vi "Get SLSC Modules By GUID.vi"(8 "error in (no error)":errorcluster, 10 "GUID":string, 11 "SLSC Chassis":u64) -> (0 "error out":errorcluster, 1 "Found":bool, 2 "SLSC Modules":u64[](array[numeric]), 3 "SLSC Chassis out":u64)   [LabVIEW 2017, in "VeriStand SLSC Scripting.lvlib"]
uses:
  VeriStand SLSC Scripting.lvlib
  NationalInstruments.VeriStand.SystemDefinitionAPI
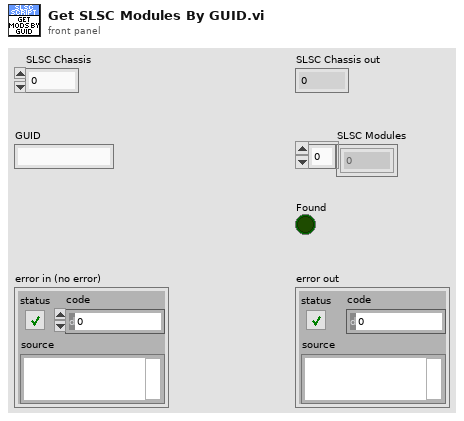
[diagram p1: front panel]
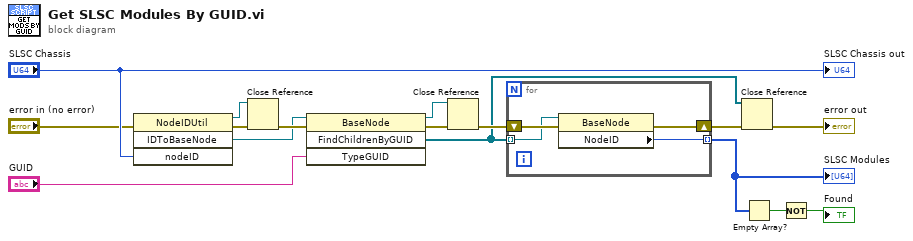
[diagram p0: block diagram]
diagram:
  n1 = invoke class="NodeIDUtil" method="IDToBaseNode"(error in="error in (no error)", "nodeID"="SLSC Chassis") -> (reference out=w15:refnum<k24>, error out=w16:errorcluster, "IDToBaseNode"=w8:refnum<k24>)  [unwired: 2 in, 1 out]
  n2 = Close Reference(reference=w15, error in (no error)=w16) -> (error out=w9:errorcluster)
  n3 = invoke class="BaseNode" method="FindChildrenByGUID"(reference=w8, error in=w9, "TypeGUID"="GUID") -> (reference out=w5:refnum<k24>, error out=w6:errorcluster, "FindChildrenByGUID"=w4:refnum<k24>[])  [unwired: 1 in, 1 out]
  n4 = Close Reference(reference=w5, error in (no error)=w6) -> (error out=w12:errorcluster)
  n5 = for {
    shift-right: [w19] -> w11
    shift-left: w12 -> [w20]
    tunnel: w4 -> [w18] mode=indexing
    tunnel: [w17] -> w3 mode=indexing
    n6 = property class="BaseNode"(reference=w18, error in=w20) -> (error out=w19:errorcluster, "NodeID"=w17:u64)  [unwired: 1 out]
  }
  "SLSC Modules" <- w3
  n7 = Close Reference(reference=w4, error in (no error)=w11) -> (error out=→"error out":errorcluster)
  n8 = Empty Array?(array=w3) -> (empty?=w2:bool)
  n9 = Not(x=w2) -> (.not. x?=→"Found":bool)
  "SLSC Chassis out" <- "SLSC Chassis"
